vi "Read Lines.vi"(8 "error in (no error)":errorcluster, 11 "user control module configuration in":refnum<class "user control module configuration.lvclass">) -> (0 "error out":errorcluster, 2 "Lines":T1(array[cluster]), 3 "user control module configuration out":refnum<class "user control module configuration.lvclass">)   [LabVIEW 2013, in "user control module configuration.lvclass"]
uses:
  user control module configuration.lvclass
  <vilib>/NI/Tag Bus Module Framework/channel/TBM channel.lvclass
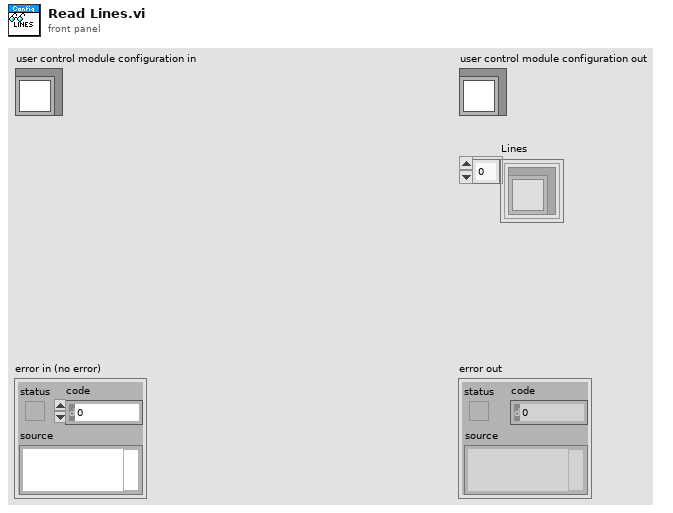
[diagram p1: front panel]
types:
  T1 = cluster{"channel":refnum<class "TBM channel.lvclass">}[]
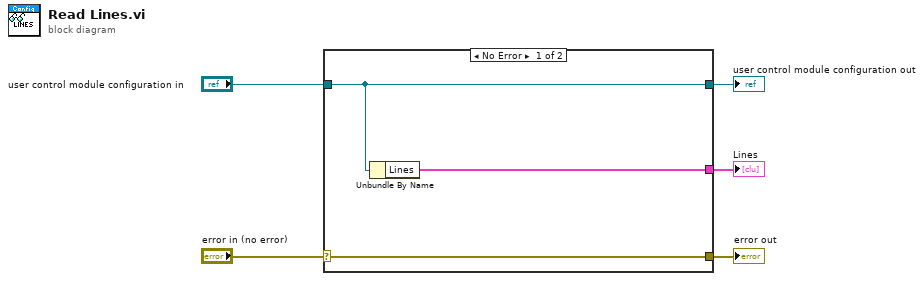
[diagram p0: block diagram]
diagram:
  n1 = case shown="No Error" "error in (no error)" {
    selector: "error in (no error)" -> [w8 w9]
    tunnel: [w8 w9] -> w4
    tunnel: [w7 w10] -> w2
    tunnel: "user control module configuration in" -> [w7 w10]
    tunnel: [w6 _] -> w1
    frame No Error {
      n2 = Unbundle By Name(w7) -> ("Lines"=w6:T1)
    }
    frame Error {
    }
  }
  "error out" <- w4
  "user control module configuration out" <- w2
  "Lines" <- w1
